vi "Gobang_getScore.vi"(1 "Position":cluster{"Cols":i32, "Rows":i32}, 2 "Color":T1, 3 "Topo":T1[][](array[typedef])) -> (0 "Score":i32)   [LabVIEW 2019, in "¤­¤l´Ñ.lvlib"]
uses:
  Piece.ctl
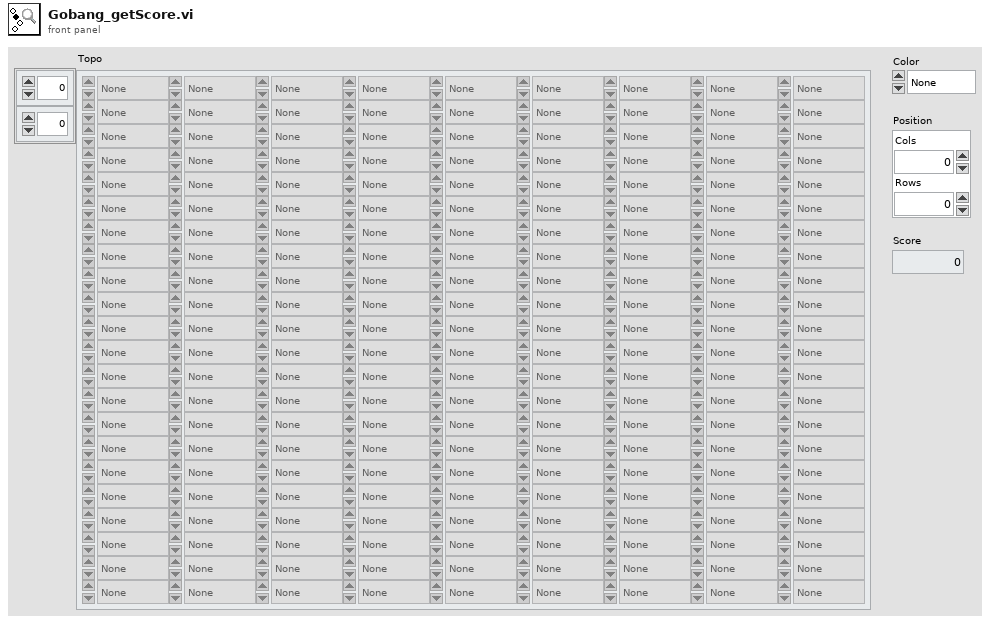
[diagram p1: front panel]
types:
  T1 = typedef "¤­¤l´Ñ.lvlib/Piece.ctl" = enum16{"None", "Black", "White"}
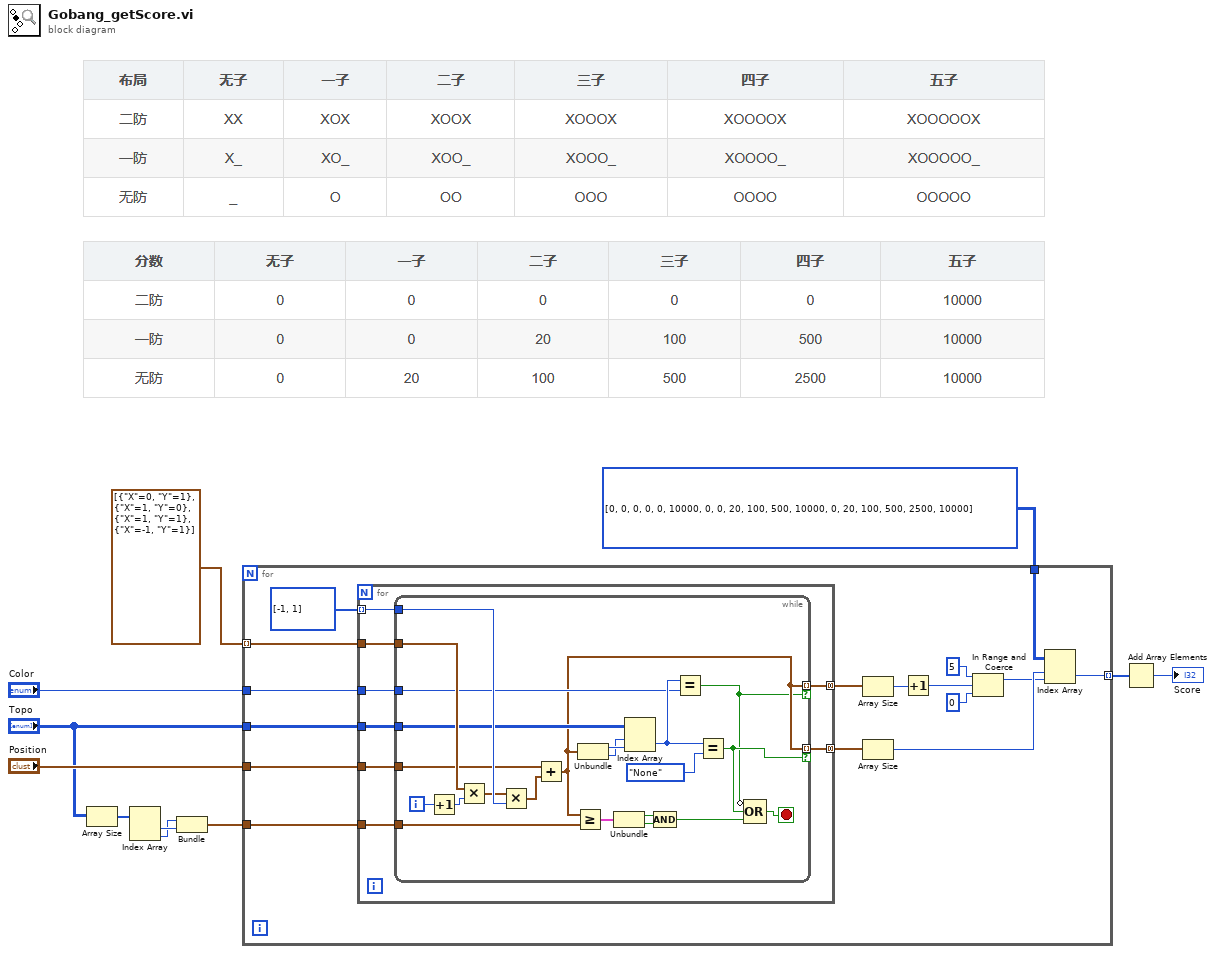
[diagram p0: block diagram]
diagram:
  n1 = Array Size(array="Topo") -> (size(s)=w8:i32[])
  n2 = Index Array(array=w8) -> (element #1=w7:i32, element #2=w6:i32)  [unwired: 2 in]
  n3 = Bundle(w6, w7) -> (w5:cluster{i32, i32})  [unwired: 1 in]
  n4 = for {
    tunnel: cluster{"X":i32, "Y":i32}[] [{"X"=0, "Y"=1}, {"X"=1, "Y"=0}, {"X"=1, "Y"=1}, {"X"=-1, "Y"=1}] -> [w27] mode=indexing
    tunnel: "Topo" -> [w26]
    tunnel: "Position" -> [w25]
    tunnel: w5 -> [w24]
    tunnel: "Color" -> [w23]
    tunnel: i32[][] [[0, 0, 0, 0, 0, 10000], [0, 0, 20, 100, 500, 10000], [0, 20, 100, 500, 2500, 10000]] -> [w19]
    tunnel: [w18] -> w2 mode=indexing
    n5 = for {
      tunnel: w27 -> [w35]
      tunnel: w26 -> [w34]
      tunnel: w25 -> [w33]
      tunnel: w24 -> [w32]
      tunnel: w23 -> [w31]
      tunnel: [w30] -> w15 mode=concatenating
      tunnel: [w29] -> w14 mode=concatenating
      tunnel: i32[] [-1, 1] -> [w28] mode=indexing
      n6 = while {
        tunnel: w35 -> [w56]
        tunnel: w34 -> [w55]
        tunnel: w33 -> [w54]
        tunnel: w32 -> [w51]
        tunnel: w31 -> [w44]
        tunnel: [w39] -> w30 mode=indexing if=w36
        tunnel: [w39] -> w29 mode=indexing if=w38
        tunnel: w28 -> [w57]
        i -> [w41]
        stop <- w46 stop-if-true
        n7 = Increment(x=w41) -> (x+1=w40:i32)
        n8 = Multiply(x=w56, y=w40) -> (x*y=w43:cluster{"X":i32, "Y":i32})
        n9 = Multiply(x=w43, y=w57) -> (x*y=w42:cluster{"X":i32, "Y":i32})
        n10 = Add(x=w54, y=w42) -> (x+y=w39:cluster{i32, i32})
        n11 = Greater Or Equal?(x=w39, y=w51) -> (x >= y?=w50:cluster{bool, bool})
        n12 = Unbundle(w39) -> (w53:i32, w52:i32)
        n13 = Unbundle(w50) -> (w49:bool, w48:bool)
        n14 = Index Array(array=w55, index (row)=w52, index (col)=w53) -> (element=w45:T1)
        n15 = Compound Arithmetic op=AND(w49, w48) -> (w37:bool)
        n16 = Equal?(x=w45, y=w44) -> (x = y?=w36:bool)
        n17 = Equal?(x=w45, y=Piece."None") -> (x = y?=w38:bool)
        n18 = Compound Arithmetic op=OR(invert w36, w38, w37) -> (w46:bool)
      }
    }
    n19 = Array Size(array=w15) -> (size(s)=w13:i32)
    n20 = Array Size(array=w14) -> (size(s)=w17:i32)
    n21 = Increment(x=w13) -> (x+1=w12:i32)
    n22 = In Range and Coerce(upper limit=5, x=w12, lower limit=0 ("upper limit")) -> (coerced(x)=w16:i32)  [unwired: 1 out]
    n23 = Index Array(array=w19, index (row)=w17, index (col)=w16) -> (element=w18:i32)
  }
  n24 = Add Array Elements(numeric array=w2) -> (sum=→"Score":i32)
